vi "Everything.vi"() -> ()   [LabVIEW 2013]
uses:
  Version Token.ctl
  APU/Settings.ctl
  APU/Input.ctl
  APU/Output.ctl
  APU/Shared Settings.ctl
  Analog Replay/Settings.ctl
  Analog Replay/Input.ctl
  Analog Replay/Load Input.ctl
  Digital Pattern Generation/Load Input.ctl
  Digital Pattern Generation/Settings.ctl
  Digital Pattern Generation/Input.ctl
  ECU Event/Timing/Measure Output.ctl
  ECU Event/Timing/Measure Settings.ctl
  ECU Event/Timing/Capture Output.ctl
  Knock Sensor/Generate Input.ctl
  Knock Sensor/Cylinder Input.ctl
  Knock Sensor/Cylinder Settings.ctl
  Knock Sensor/Generate Settings.ctl
  Directional Speed/Load Input.ctl
  Directional Speed/Settings.ctl
  Directional Speed/Input.ctl
  <vilib>/Platform/TimedLoop/XDataNode/timing_clust.ctl
  <vilib>/Platform/TimedLoop/XDataNode/nitl_modes.ctl
  <vilib>/Platform/TimedLoop/XDataNode/wakeup.ctl
  ECU Event/Timing/Capture Settings.ctl
  <vilib>/rvi/DataTransferAndStorage/Container/Common/niFpgaContainerGetUniqueNameForEmu.vi
  <vilib>/rvi/DataTransferAndStorage/Container/Common/niFpgaContainerSetEmuInfo.vi
  <vilib>/rvi/eio/common/nirviEmuReportErrorAndStop.vi
  <vilib>/rvi/Emulation/niFpgaSctlEmulationGetInTimedLoop.vi
  <vilib>/rvi/Emulation/niFpgaEmulationReportErrorSimple.vi
  <vilib>/rvi/Emulation/niFpgaGetClockAttributes.vi
  <vilib>/rvi/Emulation/niFpgaCriticalErrorInLSC.vi
  <vilib>/rvi/eio/common/nirviEmuTemplateMethod_errors.vi
  ECU Event/Timing/Measure Events (40MHz).vi
  <vilib>/Platform/TimedLoop/XDataNode/XDataNode.xnode
  <vilib>/rvi/LocalResourceManager/LocalResourceManager.xnode
  <vilib>/eio/EIONode/EIONode.xnode
  APU/APU.lvlib
  <vilib>/Platform/TimedLoop/XDataNode/XDNodeRunTimeDep.lvlib
  Analog Replay/Analog Replay.lvlib
  Digital Pattern Generation/Digital Pattern Generation.lvlib
  ECU Event/Timing/ECU Event Timing.lvlib
  Knock Sensor/Knock Sensor.lvlib
  Directional Speed/Directional Speed.lvlib
  Engine Simulation Toolkit.lvlib
panel:
  in  "go.apu 1":bool
  in  "load input.Dir Speed DIO0":T1
  in  "input.Dir Speed DIO0":T2
  in  "settings.Dir Speed DIO0":T3
  in  "input.Dir Speed DIO1":T2
  in  "settings.Dir Speed DIO1":T3
  in  "load input.Dir Speed DIO1":T1
  in  "settings.Knock AO 3":T4
  in  "settings.Knock AO 3.Cylinder 1":T5
  in  "settings.Knock AO 3.Cylinder 2":T5
  in  "settings.Knock AO 3.Cylinder 3":T5
  in  "settings.Knock AO 3.Cylinder 4":T5
  in  "input.Knock AO 3.Cylinder 1":T6
  in  "input.Knock AO 3.Cylinder 2":T6
  in  "input.Knock AO 3.Cylinder 3":T6
  in  "input.Knock AO 3.Cylinder 4":T6
  in  "input.Knock AO 3":T7
  in  "settings.Knock AO 3.Cylinder 5":T5
  in  "settings.Knock AO 3.Cylinder 6":T5
  in  "input.Knock AO 3.Cylinder 5":T6
  in  "input.Knock AO 3.Cylinder 6":T6
  in  "settings.Knock AO 2.Cylinder 5":T5
  in  "settings.Knock AO 2.Cylinder 6":T5
  in  "input.Knock AO 2.Cylinder 5":T6={"probability compare"=65535, "high freq scaler"=0.0, "trigger position"=0}
  in  "input.Knock AO 2.Cylinder 6":T6={"probability compare"=65535, "high freq scaler"=0.0, "trigger position"=0}
  in  "settings.Knock AO 2":T4
  in  "settings.Knock AO 2.Cylinder 1":T5
  in  "settings.Knock AO 2.Cylinder 2":T5
  in  "settings.Knock AO 2.Cylinder 3":T5
  in  "settings.Knock AO 2.Cylinder 4":T5
  in  "input.Knock AO 2.Cylinder 1":T6={"probability compare"=65535, "high freq scaler"=0.0, "trigger position"=0}
  in  "input.Knock AO 2.Cylinder 2":T6={"probability compare"=65535, "high freq scaler"=0.0, "trigger position"=0}
  in  "input.Knock AO 2.Cylinder 3":T6={"probability compare"=65535, "high freq scaler"=0.0, "trigger position"=0}
  in  "input.Knock AO 2.Cylinder 4":T6={"probability compare"=65535, "high freq scaler"=0.0, "trigger position"=0}
  in  "input.Knock AO 2":T7
  out "capture.Multi Event DIO 15.Event 4":T8
  out "capture.Multi Event DIO 15.Event 3":T8
  out "capture.Multi Event DIO 15.Event 2":T8
  out "capture.Multi Event DIO 14.Event 4":T8
  out "capture.Multi Event DIO 14.Event 3":T8
  out "capture.Multi Event DIO 14.Event 2":T8
  out "capture.Multi Event DIO 13.Event 4":T8
  out "capture.Multi Event DIO 13.Event 3":T8
  out "capture.Multi Event DIO 13.Event 2":T8
  out "capture.Multi Event DIO 12.Event 4":T8
  out "capture.Multi Event DIO 12.Event 3":T8
  out "capture.Multi Event DIO 12.Event 2":T8
  out "capture.Multi Event DIO 11.Event 4":T8
  out "capture.Multi Event DIO 11.Event 3":T8
  out "capture.Multi Event DIO 11.Event 2":T8
  out "capture.Multi Event DIO 10.Event 4":T8
  out "capture.Multi Event DIO 10.Event 3":T8
  out "capture.Multi Event DIO 10.Event 2":T8
  out "capture.Multi Event DIO 10.Event 1":T8
  out "capture.Multi Event DIO 11.Event 1":T8
  out "capture.Multi Event DIO 12.Event 1":T8
  out "capture.Multi Event DIO 13.Event 1":T8
  out "capture.Multi Event DIO 14.Event 1":T8
  out "capture.Multi Event DIO 15.Event 1":T8
  in  "settings.Multi Event DIO 10":T9
  in  "settings.Multi Event DIO 11":T9
  in  "settings.Multi Event DIO 12":T9
  in  "settings.Multi Event DIO 13":T9
  in  "settings.Multi Event DIO 14":T9
  in  "settings.Multi Event DIO 15":T9
  out "status.Multi Event DIO 10":T10
  out "status.Multi Event DIO 11":T10
  out "status.Multi Event DIO 12":T10
  out "status.Multi Event DIO 13":T10
  out "status.Multi Event DIO 14":T10
  out "status.Multi Event DIO 15":T10
  out "capture.Event DIO 4.Event 1":T8
  out "capture.Event DIO 5.Event 1":T8
  out "capture.Event DIO 6.Event 1":T8
  out "capture.Event DIO 7.Event 1":T8
  out "capture.Event DIO 8.Event 1":T8
  out "capture.Event DIO 9.Event 1":T8
  in  "settings.Event DIO 4":T9
  in  "settings.Event DIO 5":T9
  in  "settings.Event DIO 6":T9
  in  "settings.Event DIO 7":T9
  in  "settings.Event DIO 8":T9
  in  "settings.Event DIO 9":T9
  out "status.Event DIO 4":T10
  out "status.Event DIO 5":T10
  out "status.Event DIO 6":T10
  out "status.Event DIO 7":T10
  out "status.Event DIO 8":T10
  out "status.Event DIO 9":T10
  in  "load input.Pattern DIO 3":T11
  in  "load input.Pattern DIO 2":T11
  in  "load input.Pattern DIO 1":T11
  in  "input.Pattern DIO 0":T12
  in  "settings.Pattern DIO 0":T13
  in  "input.Pattern DIO 1":T12
  in  "settings.Pattern DIO 1":T13
  in  "input.Pattern DIO 2":T12
  in  "settings.Pattern DIO 2":T13
  in  "input.Pattern DIO 3":T12
  in  "settings.Pattern DIO 3":T13
  in  "load input.Pattern DIO 0":T11
  in  "load input.replay AO 1":T14={"Data"=[0, 0, 0, 0, 0, 0, 0, 0, 0, 0, 0, 0, 0, 0, 0, 0], "LoadOffset"=0, "Done"=FALSE} caption="input"
  in  "load input.replay AO 0":T14={"Data"=[0, 0, 0, 0, 0, 0, 0, 0, 0, 0, 0, 0, 0, 0, 0, 0], "LoadOffset"=0, "Done"=FALSE} caption="input"
  in  "input.replay AO 0":T15 caption="input"
  in  "input.replay AO 1":T15 caption="input"
  in  "settings.replay AO 1":T16 caption="settings"
  in  "settings.replay AO 0":T16 caption="settings"
  in  "shared settings.apu 1":T17 {"start" format="%#.15g"}
  out "output.apu 1":T18 caption="output"
  in  "input.apu 1":T19={"desired speed"=0.0, "reset"=TRUE} caption="input"
  in  "settings.apu 1":T20 caption="settings"
  in  "est.version":T21
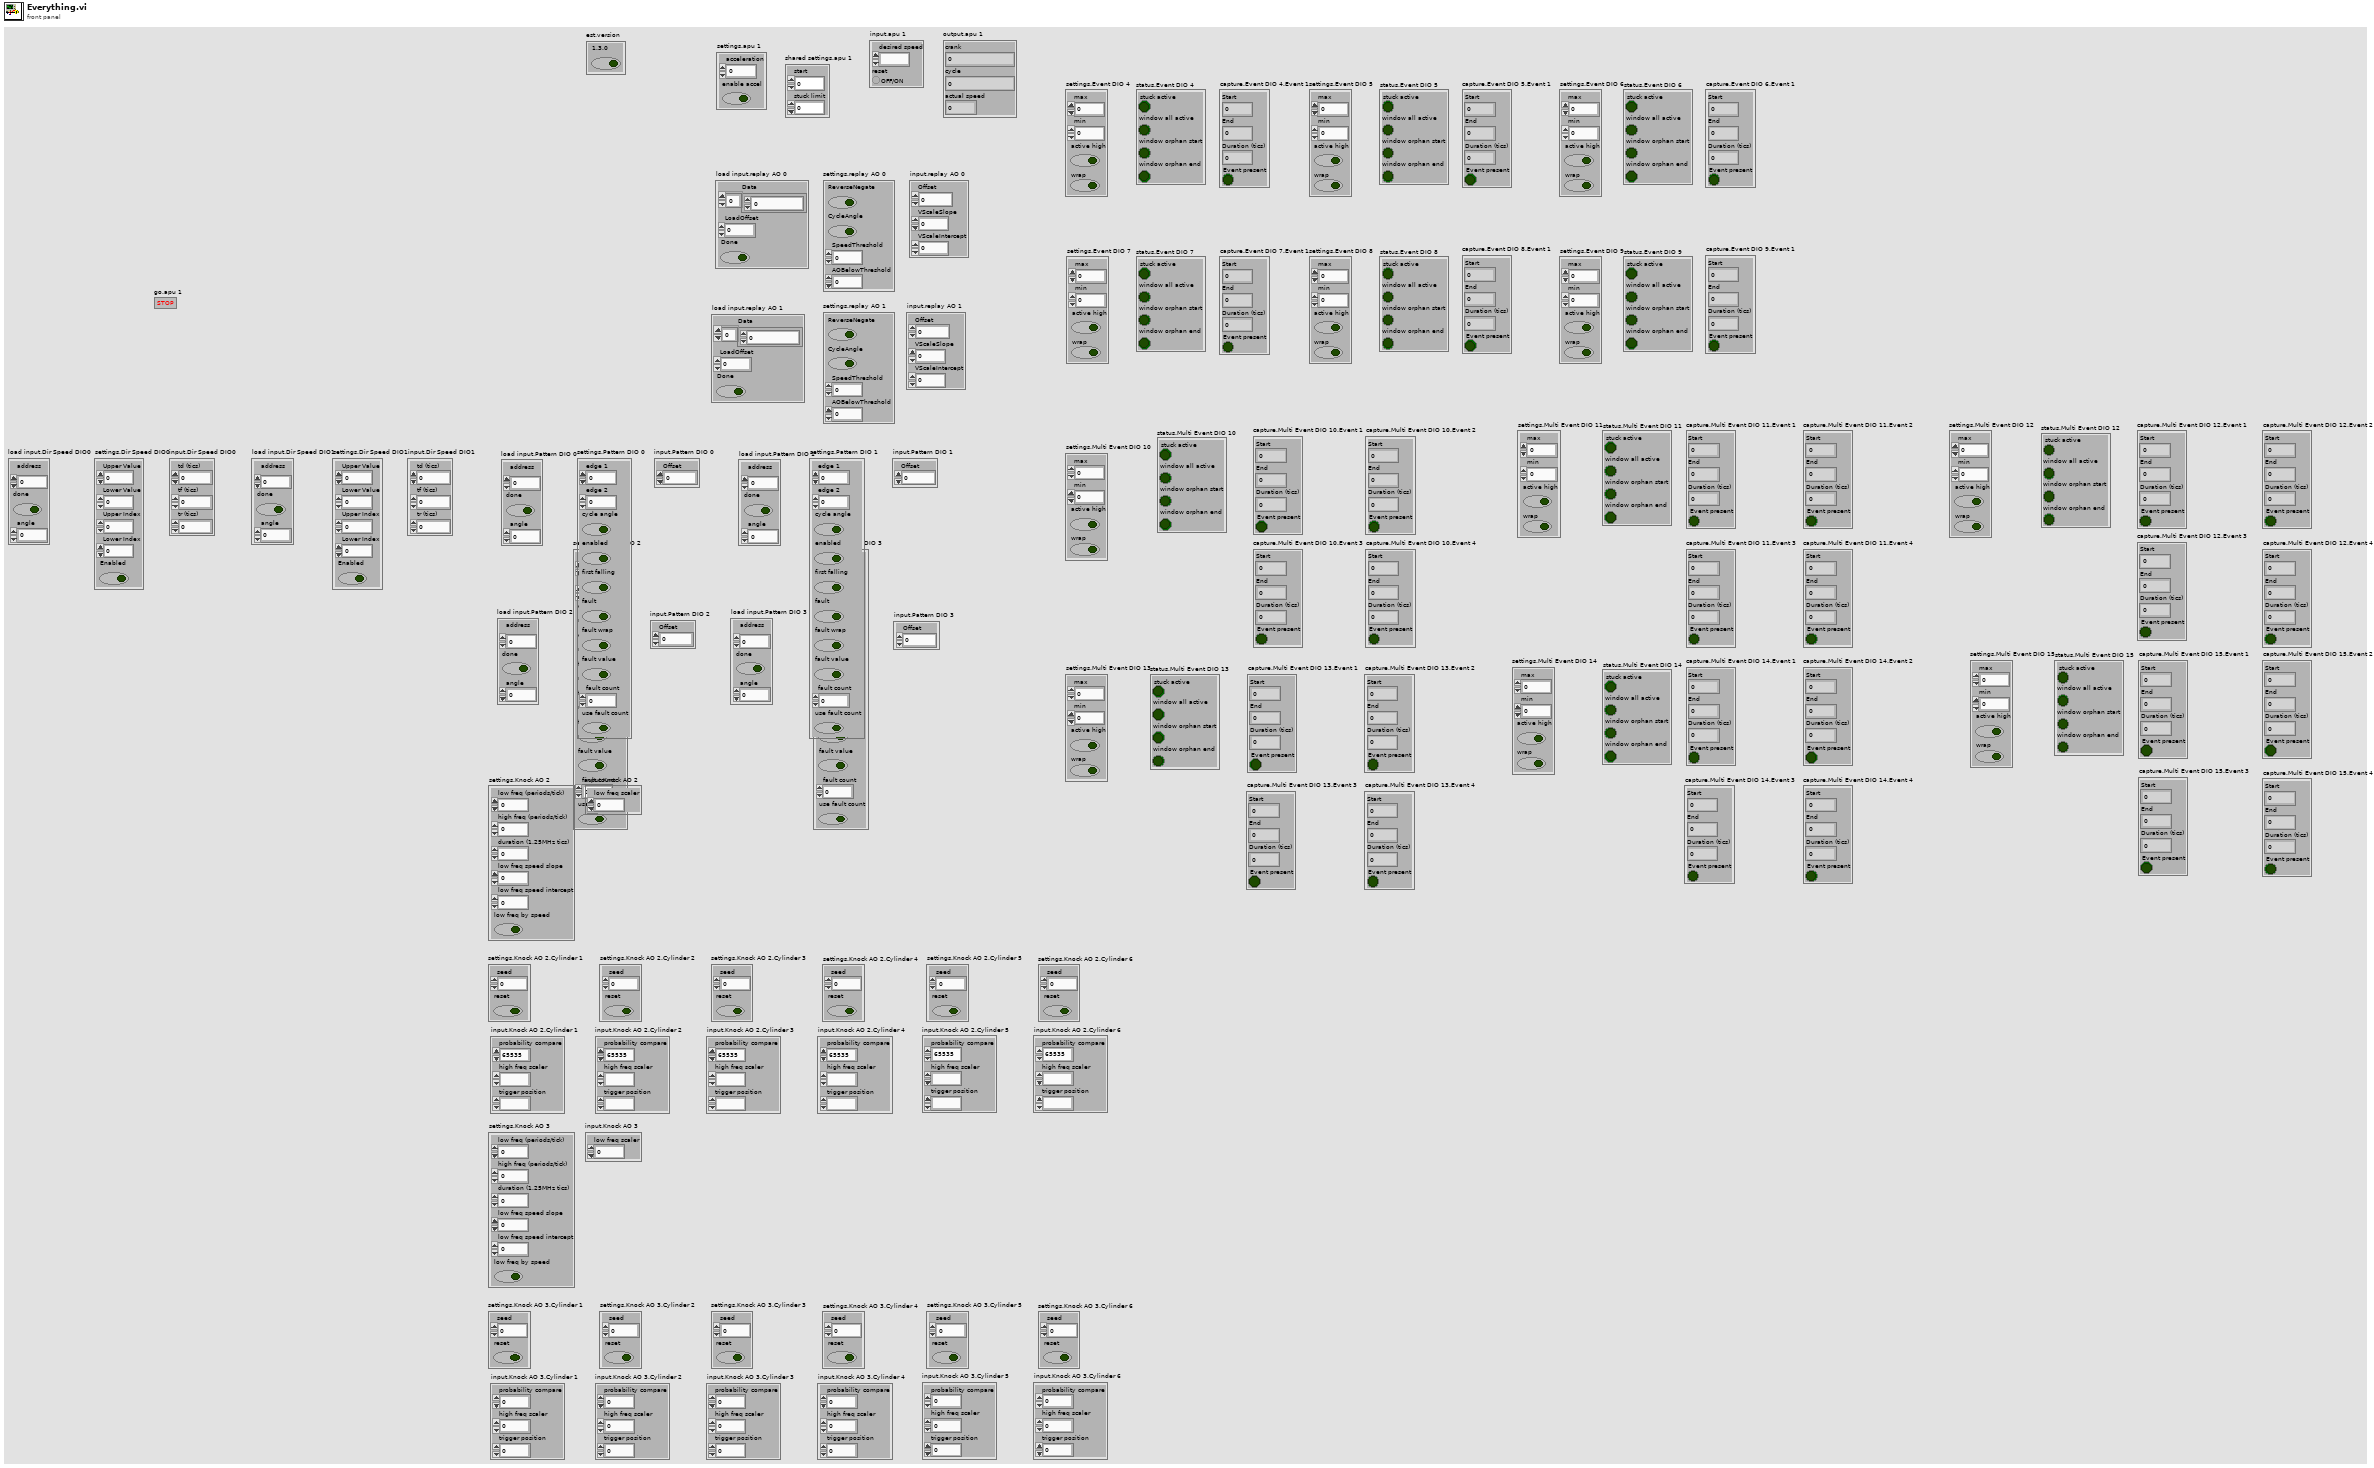
[diagram p1: front panel]
types:
  T1 = typedef "Engine Simulation Toolkit.lvlib/Directional Speed.lvlib/Load Input.ctl" = cluster{"address":fxp<+,10,10>, "done":bool, "angle":u16}
  T2 = typedef "Engine Simulation Toolkit.lvlib/Directional Speed.lvlib/Input.ctl" = cluster{"td (tics)":u16, "tf (tics)":u16, "tr (tics)":u16}
  T3 = typedef "Engine Simulation Toolkit.lvlib/Directional Speed.lvlib/Settings.ctl" = cluster{"Upper Value":u16, "Lower Value":u16, "Upper Index":fxp<+,10,10>, "Lower Index":fxp<+,10,10>, "Enabled":bool}
  T4 = typedef "Engine Simulation Toolkit.lvlib/Knock Sensor.lvlib/Generate Settings.ctl" = cluster{"low freq (periods/tick)":fxp<+,32,0>, "high freq (periods/tick)":fxp<+,32,0>, "duration (1.25MHz tics)":fxp<+,18,18>, "low freq speed slope":fxp<+,16,-3>, "low freq speed intercept":fxp<+,10,-10>, "low freq by speed":bool}
  T5 = typedef "Engine Simulation Toolkit.lvlib/Knock Sensor.lvlib/Cylinder Settings.ctl" = cluster{"seed":u16, "reset":bool}
  T6 = typedef "Engine Simulation Toolkit.lvlib/Knock Sensor.lvlib/Cylinder Input.ctl" = cluster{"probability compare":u16, "high freq scaler":fxp<+,10,0>, "trigger position":u16}
  T7 = typedef "Engine Simulation Toolkit.lvlib/Knock Sensor.lvlib/Generate Input.ctl" = cluster{"low freq scaler":fxp<+,10,0>}
  T8 = typedef "Engine Simulation Toolkit.lvlib/ECU Event Timing.lvlib/Capture Output.ctl" = cluster{"Start":u16, "End":u16, "Duration (tics)":fxp<+,18,18>, "Event present":bool}
  T9 = typedef "Engine Simulation Toolkit.lvlib/ECU Event Timing.lvlib/Measure Settings.ctl" = cluster{"max":u16, "min":u16, "active high":bool, "wrap":bool}
  T10 = typedef "Engine Simulation Toolkit.lvlib/ECU Event Timing.lvlib/Measure Output.ctl" = cluster{"stuck active":bool, "window all active":bool, "window orphan start":bool, "window orphan end":bool}
  T11 = typedef "Engine Simulation Toolkit.lvlib/Digital Pattern Generation.lvlib/Load Input.ctl" = cluster{"address":fxp<+,11,11>, "done":bool, "angle":u16}
  T12 = typedef "Engine Simulation Toolkit.lvlib/Digital Pattern Generation.lvlib/Input.ctl" = cluster{"Offset":i16}
  T13 = typedef "Engine Simulation Toolkit.lvlib/Digital Pattern Generation.lvlib/Settings.ctl" = cluster{"edge 1":u16, "edge 2":u16, "cycle angle":bool, "enabled":bool, "first falling":bool, "fault":bool, "fault wrap":bool, "fault value":bool, "fault count":fxp<+,4,4>, "use fault count":bool}
  T14 = typedef "Engine Simulation Toolkit.lvlib/Analog Replay.lvlib/Load Input.ctl" = cluster{"Data":i16[], "LoadOffset":u16, "Done":bool}
  T15 = typedef "Engine Simulation Toolkit.lvlib/Analog Replay.lvlib/Input.ctl" = cluster{"Offset":i16, "VScaleSlope":fxp<+,18,6>, "VScaleIntercept":fxp<+/-,18,3>}
  T16 = typedef "Engine Simulation Toolkit.lvlib/Analog Replay.lvlib/Settings.ctl" = cluster{"ReverseNegate":bool, "CycleAngle":bool, "SpeedThreshold":fxp<+/-,23,2>, "AOBelowThreshold":i16}
  T17 = typedef "Engine Simulation Toolkit.lvlib/APU.lvlib/Shared Settings.ctl" = cluster{"start":fxp<+,17,17>, "stuck limit":fxp<+,18,18>}
  T18 = typedef "Engine Simulation Toolkit.lvlib/APU.lvlib/Output.ctl" = cluster{"crank":u16, "cycle":u16, "actual speed":fxp<+/-,23,2>}
  T19 = typedef "Engine Simulation Toolkit.lvlib/APU.lvlib/Input.ctl" = cluster{"desired speed":fxp<+/-,23,2>, "reset":bool}
  T20 = typedef "Engine Simulation Toolkit.lvlib/APU.lvlib/Settings.ctl" = cluster{"acceleration":fxp<+,18,-20>, "enable accel":bool}
  T21 = typedef "Engine Simulation Toolkit.lvlib/Version Token.ctl" = cluster{"1.3.0":bool}
  T22 = typedef "XDNodeRunTimeDep.lvlib/timing_clust.ctl" = cluster{"Expected End [f-1]":u64, "Actual End [f-1]":u64, "Finished Late? [f-1]":bool, "Expected End [i-1]":u64, "Actual End [i-1]":u64, "Finished Late? [i-1]":bool, "Expected Start [i]":u64, "Actual Start [i]":u64, "Expected Start [f]":u64, "Actual Start [f]":u64, "Source Name":string, "Structure Name":string, "Period":i64, "Deadline":i64, "Offset":i64, "Start":i64, "Priority":i32, "Timeout":i32, "Mode":T23, "Wakeup Reason":T24, "Error":errorcluster, "Source Type":string, "Secondary Source Type":string, "Global End Time":u64, "Global Start Time":u64, "Frame Duration":u64, "Iteration Duration":u64, "Assigned CPU":i32, "I/O Scan Engine Mode":u32}
  T23 = typedef "XDNodeRunTimeDep.lvlib/nitl_modes.ctl" = enum32{"No Change", "Process missed periods, maintain original phase", "Discard missed periods, maintain original phase", "Process missed periods, ignore original phase", "Discard missed periods, ignore original phase"}
  T24 = typedef "XDNodeRunTimeDep.lvlib/wakeup.ctl" = enum32{"Normal", "Aborted", "Asynchronous wakeup", "Timing source error", "Timed loop error", "Timeout"}
  T25 = typedef "Engine Simulation Toolkit.lvlib/Directional Speed.lvlib/Load Data.ctl" = cluster{"max address":fxp<+,10,10>, "Memory":refnum<k21>}
  T26 = typedef "Engine Simulation Toolkit.lvlib/APU.lvlib/Register Bus.ctl" = cluster{"Speed":refnum<k21>, "Crank Angle":refnum<k21>, "Cycle Angle":refnum<k21>, "Crank Count":refnum<k21>, "Cycle Count":refnum<k21>, "1.25 MHz Counter":refnum<k21>, "Crank Rollover":refnum<k21>, "Cycle Rollover":refnum<k21>, "shared settings":T17}
  T27 = typedef "Engine Simulation Toolkit.lvlib/Digital Pattern Generation.lvlib/Load Data.ctl" = cluster{"max address":fxp<+,11,11>, "memory":refnum<k21>}
  T28 = typedef "Engine Simulation Toolkit.lvlib/Knock Sensor.lvlib/Triggered Cylinder Data.ctl" = cluster{"trigger knock":bool, "high freq scaler":fxp<+,10,0>}
  T29 = typedef "Engine Simulation Toolkit.lvlib/ECU Event Timing.lvlib/Capture Settings.ctl" = u8
  T30 = typedef "Engine Simulation Toolkit.lvlib/ECU Event Timing.lvlib/Measured Data.ctl" = cluster{"start":u16, "end":u16, "duration (tics)":fxp<+,18,18>, "window end":bool, "window begin":bool, "pulse end":bool, "pulse #":u8}
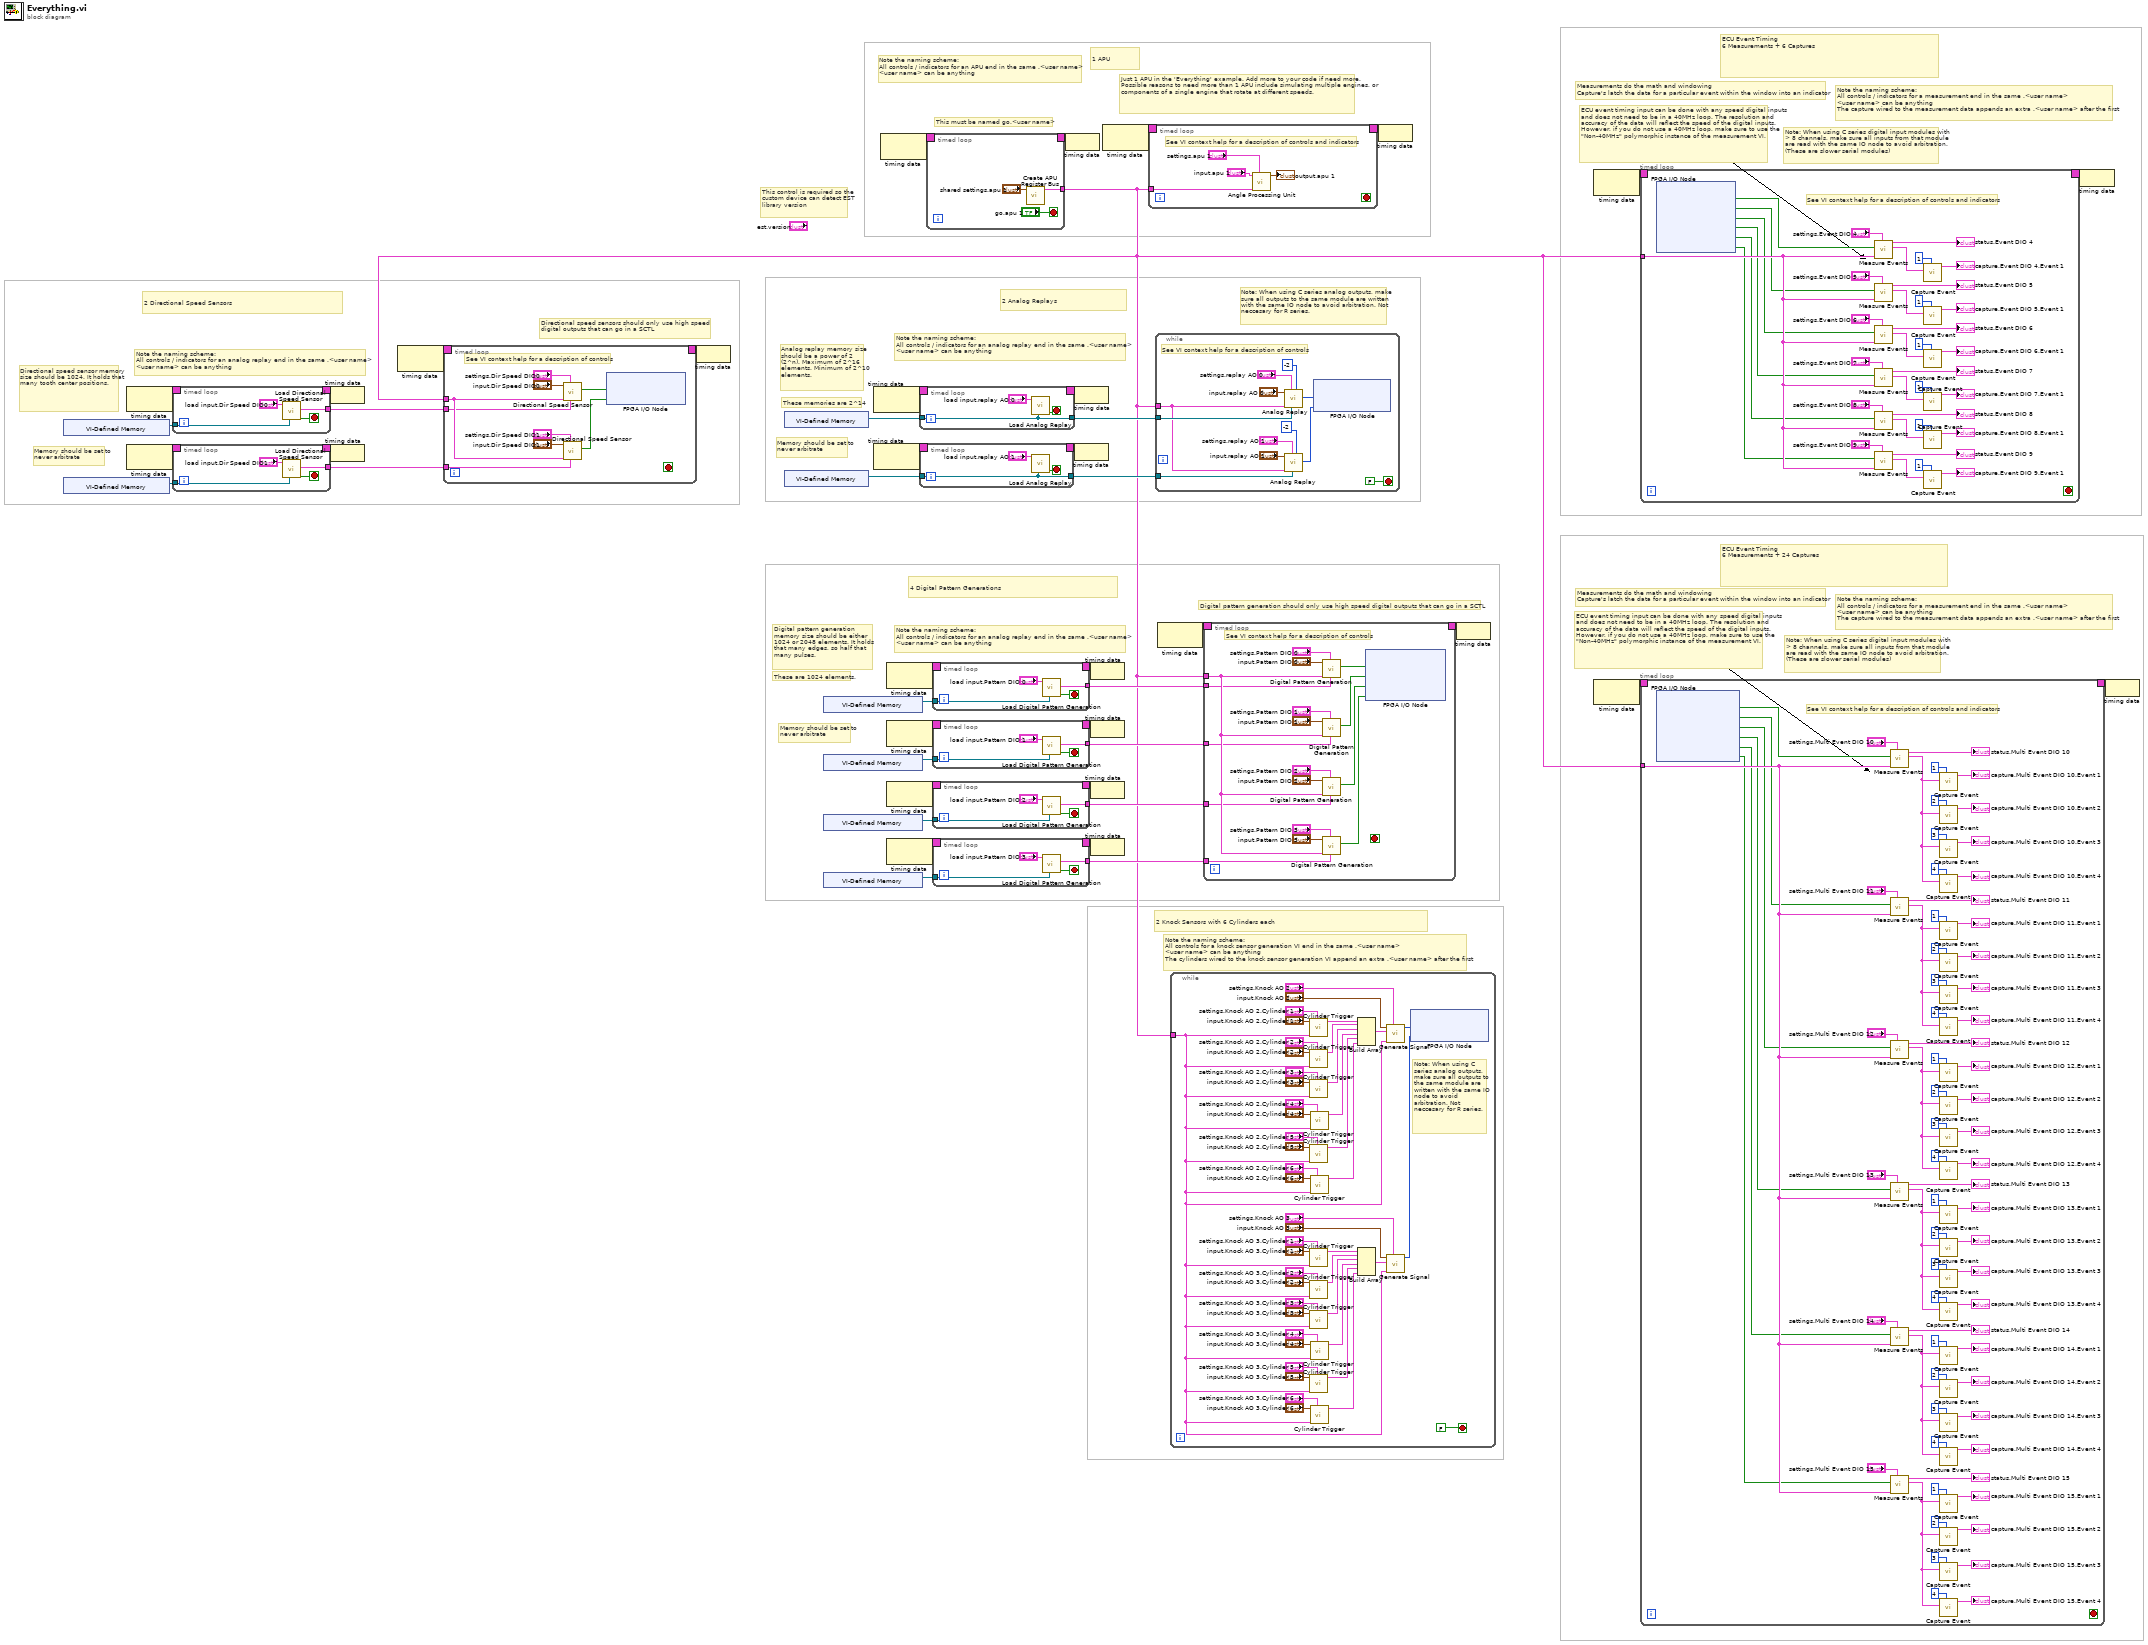
[diagram p0: block diagram]
diagram:
  # "ECU event timing input can be done with any speed digital inputs and does not need to be in a 40MHz loop. The resolution and accuracy of the data will reflect the speed of the digital inputs. However, if you do not use a 40MHz loop, make sure to use the \"Non-40MHz\" polymorphic instance of the measurement VI."
  # "This must be named go.<user name>"
  # "Memory should be set to never arbitrate"
  # "Memory should be set to never arbitrate"
  # "Memory should be set to never arbitrate"
  # "Note the naming scheme: \nAll controls / indicators for an analog replay end in the same .<user name>\n<user name> can be anything"
  # "Directional speed sensor memory size should be 1024. It holds that many tooth center positions."
  # "Directional speed sensors should only use high speed digital outputs that can go in a SCTL"
  # "2 Directional Speed Sensors"
  # "Note the naming scheme: \nAll controls for a knock sensor generation VI end in the same .<user name>\n<user name> can be anything\nThe cylinders wired to the knock sensor generation VI append an extra .<user name> after the first"
  # "2 Knock Sensors with 6 Cylinders each"
  # "Note: When using C series digital input modules with > 8 channels, make sure all inputs from that module are read with the same IO node to avoid arbitration. (These are slower serial modules)"
  # "Measurements do the math and windowing\nCapture's latch the data for a particular event within the window into an indicator"
  # "ECU Event Timing\n6 Measurements + 24 Captures"
  # "Note the naming scheme: \nAll controls / indicators for a measurement end in the same .<user name>\n<user name> can be anything\nThe capture wired to the measurement data appends an extra .<user name> after the first"
  # "Note: When using C series digital input modules with > 8 channels, make sure all inputs from that module are read with the same IO node to avoid arbitration. (These are slower serial modules)"
  # "Measurements do the math and windowing\nCapture's latch the data for a particular event within the window into an indicator"
  # "ECU Event Timing\n6 Measurements + 6 Captures"
  # "Note the naming scheme: \nAll controls / indicators for a measurement end in the same .<user name>\n<user name> can be anything\nThe capture wired to the measurement data appends an extra .<user name> after the first"
  # "ECU event timing input can be done with any speed digital inputs and does not need to be in a 40MHz loop. The resolution and accuracy of the data will reflect the speed of the digital inputs. However, if you do not use a 40MHz loop, make sure to use the \"Non-40MHz\" polymorphic instance of the measurement VI."
  # "Digital pattern generation should only use high speed digital outputs that can go in a SCTL"
  # "4 Digital Pattern Generations"
  # "Note the naming scheme: \nAll controls / indicators for an analog replay end in the same .<user name>\n<user name> can be anything"
  # "These are 1024 elements."
  # "Digital pattern generation memory size should be either 1024 or 2048 elements. It holds that many edges, so half that many pulses."
  # "Note: When using C series analog outputs, make sure all outputs to the same module are written with the same IO node to avoid arbitration. Not neccesary for R series."
  # "2 Analog Replays"
  # "1 APU"
  # "These memories are 2^14"
  # "Note the naming scheme: \nAll controls / indicators for an APU end in the same .<user name>\n<user name> can be anything"
  # "Note the naming scheme: \nAll controls / indicators for an analog replay end in the same .<user name>\n<user name> can be anything"
  # "Analog replay memory size should be a power of 2 (2^n). Maximum of 2^16 elements. Minimum of 2^10 elements."
  # "Just 1 APU in the 'Everything' example. Add more to your code if need more. Possible reasons to need more than 1 APU include simulating multiple engines, or components of a single engine that rotate at different speeds."
  # "This control is required so the custom device can detect EST library version"
  n1 = xnode "VI-Defined Memory"() -> ("Memory Out"=w4:refnum<k21>)
  n2 = xnode "VI-Defined Memory"() -> ("Memory Out"=w6:refnum<k21>)
  n3 = node-c288() -> (w13:T22)  [unwired: 1 in]
  n4 = node-c288() -> (w9:T22)  [unwired: 1 in]
  n5 = timed-loop {
    timing: w13 -> [_]
    timing-out: [_] -> w12
    tunnel: w4 -> [w48]
    tunnel: [w47] -> w5
    stop <- w49 stop-if-true
    n6 = call "Load Directional Speed Sensor.vi"("Memory In"=w48, "load input.<user name>"="load input.Dir Speed DIO0") -> ("done"=w49:bool, "load data"=w47:T25)  [unwired: 8 in]
  }
  n7 = timed-loop {
    timing: w9 -> [_]
    timing-out: [_] -> w8
    tunnel: w6 -> [w54]
    tunnel: [w53] -> w7
    stop <- w55 stop-if-true
    n8 = call "Load Directional Speed Sensor.vi"("Memory In"=w54, "load input.<user name>"="load input.Dir Speed DIO1") -> ("done"=w55:bool, "load data"=w53:T25)  [unwired: 8 in]
  }
  n9 = node-c288(w12) -> ()
  n10 = node-c288(w8) -> ()
  n11 = node-c288() -> (w11:T22)  [unwired: 1 in]
  n12 = xnode "VI-Defined Memory"() -> ("Memory Out"=w38:refnum<k21>)
  n13 = xnode "VI-Defined Memory"() -> ("Memory Out"=w39:refnum<k21>)
  n14 = xnode "VI-Defined Memory"() -> ("Memory Out"=w31:refnum<k21>)
  n15 = xnode "VI-Defined Memory"() -> ("Memory Out"=w27:refnum<k21>)
  n16 = xnode "VI-Defined Memory"() -> ("Memory Out"=w24:refnum<k21>)
  n17 = xnode "VI-Defined Memory"() -> ("Memory Out"=w21:refnum<k21>)
  n18 = node-c288() -> (w43:T22)  [unwired: 1 in]
  n19 = node-c288() -> (w41:T22)  [unwired: 1 in]
  n20 = node-c288() -> (w2:T22)  [unwired: 1 in]
  n21 = node-c288() -> (w35:T22)  [unwired: 1 in]
  n22 = node-c288() -> (w29:T22)  [unwired: 1 in]
  n23 = node-c288() -> (w26:T22)  [unwired: 1 in]
  n24 = node-c288() -> (w23:T22)  [unwired: 1 in]
  n25 = timed-loop {
    timing: w43 -> [_]
    timing-out: [_] -> w42
    tunnel: w38 -> [w58]
    tunnel: [w58] -> w37
    stop <- w59 stop-if-true
    n26 = call "Load Analog Replay.vi"("memory"=w58, "load input.<user name>"="load input.replay AO 0") -> ("done"=w59:bool)  [unwired: 9 in]
  }
  n27 = timed-loop {
    timing: w41 -> [_]
    timing-out: [_] -> w40
    tunnel: w39 -> [w63]
    tunnel: [w63] -> w36
    stop <- w64 stop-if-true
    n28 = call "Load Analog Replay.vi"("memory"=w63, "load input.<user name>"="load input.replay AO 1") -> ("done"=w64:bool)  [unwired: 9 in]
  }
  n29 = timed-loop {
    timing: w2 -> [_]
    timing-out: [_] -> w1
    tunnel: [w69] -> w3
    stop <- "go.apu 1" stop-if-true
    n30 = call "Create APU Register Bus.vi"("shared settings.<user name>"="shared settings.apu 1") -> ("register bus"=w69:T26)  [unwired: 10 in]
  }
  n31 = timed-loop {
    tunnel: w3 -> [w75]
    timing: w11 -> [_]
    timing-out: [_] -> w10
    tunnel: w5 -> [w74]
    tunnel: w7 -> [w73]
    stop <- _ stop-if-true
    # "See VI context help for a description of controls"
    n32 = call "Directional Speed Sensor.vi"("load data"=w74, "settings.<user name>"="settings.Dir Speed DIO0", "register bus"=w75, "input.<user name>"="input.Dir Speed DIO0") -> ("digial output"=w78:bool)  [unwired: 7 in]
    n33 = call "Directional Speed Sensor.vi"("load data"=w73, "settings.<user name>"="settings.Dir Speed DIO1", "register bus"=w75, "input.<user name>"="input.Dir Speed DIO1") -> ("digial output"=w79:bool)  [unwired: 7 in]
    n34 = xnode "FPGA I/O Node"("Connector1/DIO0"=w78, "Connector1/DIO1"=w79) -> ()  [unwired: 2 in, 2 out]
  }
  n35 = node-c288(w10) -> ()
  n36 = timed-loop {
    timing: w35 -> [_]
    timing-out: [_] -> w34
    tunnel: w31 -> [w86]
    tunnel: [w85] -> w30
    stop <- w87 stop-if-true
    n37 = call "Load Digital Pattern Generation.vi"("memory"=w86, "load input.<user name>"="load input.Pattern DIO 0") -> ("done"=w87:bool, "load data"=w85:T27)  [unwired: 8 in]
  }
  n38 = timed-loop {
    timing: w29 -> [_]
    timing-out: [_] -> w28
    tunnel: w27 -> [w92]
    tunnel: [w91] -> w18
    stop <- w93 stop-if-true
    n39 = call "Load Digital Pattern Generation.vi"("memory"=w92, "load input.<user name>"="load input.Pattern DIO 1") -> ("done"=w93:bool, "load data"=w91:T27)  [unwired: 8 in]
  }
  n40 = timed-loop {
    timing: w26 -> [_]
    timing-out: [_] -> w25
    tunnel: w24 -> [w98]
    tunnel: [w97] -> w19
    stop <- w99 stop-if-true
    n41 = call "Load Digital Pattern Generation.vi"("memory"=w98, "load input.<user name>"="load input.Pattern DIO 2") -> ("done"=w99:bool, "load data"=w97:T27)  [unwired: 8 in]
  }
  n42 = timed-loop {
    timing: w23 -> [_]
    timing-out: [_] -> w22
    tunnel: w21 -> [w104]
    tunnel: [w103] -> w20
    stop <- w105 stop-if-true
    n43 = call "Load Digital Pattern Generation.vi"("memory"=w104, "load input.<user name>"="load input.Pattern DIO 3") -> ("done"=w105:bool, "load data"=w103:T27)  [unwired: 8 in]
  }
  n44 = node-c288(w1) -> ()
  n45 = node-c288(w40) -> ()
  n46 = node-c288(w42) -> ()
  n47 = node-c288(w34) -> ()
  n48 = node-c288(w28) -> ()
  n49 = node-c288(w25) -> ()
  n50 = node-c288(w22) -> ()
  n51 = node-c288() -> (w45:T22)  [unwired: 1 in]
  n52 = timed-loop {
    timing: w45 -> [_]
    timing-out: [_] -> w44
    tunnel: w3 -> [w108]
    stop <- _ stop-if-true
    # "See VI context help for a description of controls and indicators"
    n53 = call "Angle Processing Unit.vi"("settings.<user name>"="settings.apu 1", "register bus"=w108, "input.<user name>"="input.apu 1") -> ("output.<user name>"=→"output.apu 1":T18)  [unwired: 8 in]
  }
  n54 = while {
    tunnel: w37 -> [w125]
    tunnel: w3 -> [w114]
    tunnel: w36 -> [w122]
    stop <- FALSE stop-if-true
    # "See VI context help for a description of controls"
    n55 = call "Analog Replay.vi"("shift"=i8 -2, "memory"=w125, "settings.<user name>"="settings.replay AO 0", "register bus"=w114, "input.<user name>"="input.replay AO 0") -> ("analog value"=w118:i16)  [unwired: 6 in]
    n56 = call "Analog Replay.vi"("shift"=i8 -2, "memory"=w122, "settings.<user name>"="settings.replay AO 1", "register bus"=w114, "input.<user name>"="input.replay AO 1") -> ("analog value"=w117:i16)  [unwired: 6 in]
    n57 = xnode "FPGA I/O Node"("Connector0/AO0"=w118, "Connector0/AO1"=w117) -> ()  [unwired: 2 in, 2 out]
  }
  n58 = node-c288() -> (w33:T22)  [unwired: 1 in]
  n59 = while {
    tunnel: w3 -> [w127]
    stop <- FALSE stop-if-true
    # "Note: When using C series analog outputs, make sure all outputs to the same module are written with the same IO node to avoid arbitration. Not neccesary for R series."
    n60 = call "Cylinder Trigger.vi"("settings.<user name>"="settings.Knock AO 2.Cylinder 1", "register bus"=w127, "input.<user name>"="input.Knock AO 2.Cylinder 1") -> ("triggered knock data"=w171:T28)  [unwired: 8 in]
    n61 = call "Cylinder Trigger.vi"("settings.<user name>"="settings.Knock AO 2.Cylinder 2", "register bus"=w127, "input.<user name>"="input.Knock AO 2.Cylinder 2") -> ("triggered knock data"=w170:T28)  [unwired: 8 in]
    n62 = call "Cylinder Trigger.vi"("settings.<user name>"="settings.Knock AO 2.Cylinder 3", "register bus"=w127, "input.<user name>"="input.Knock AO 2.Cylinder 3") -> ("triggered knock data"=w169:T28)  [unwired: 8 in]
    n63 = call "Cylinder Trigger.vi"("settings.<user name>"="settings.Knock AO 2.Cylinder 5", "register bus"=w127, "input.<user name>"="input.Knock AO 2.Cylinder 5") -> ("triggered knock data"=w150:T28)  [unwired: 8 in]
    n64 = call "Cylinder Trigger.vi"("settings.<user name>"="settings.Knock AO 3.Cylinder 1", "register bus"=w127, "input.<user name>"="input.Knock AO 3.Cylinder 1") -> ("triggered knock data"=w128:T28)  [unwired: 8 in]
    n65 = call "Cylinder Trigger.vi"("settings.<user name>"="settings.Knock AO 3.Cylinder 2", "register bus"=w127, "input.<user name>"="input.Knock AO 3.Cylinder 2") -> ("triggered knock data"=w129:T28)  [unwired: 8 in]
    n66 = call "Cylinder Trigger.vi"("settings.<user name>"="settings.Knock AO 3.Cylinder 3", "register bus"=w127, "input.<user name>"="input.Knock AO 3.Cylinder 3") -> ("triggered knock data"=w130:T28)  [unwired: 8 in]
    n67 = call "Cylinder Trigger.vi"("settings.<user name>"="settings.Knock AO 3.Cylinder 5", "register bus"=w127, "input.<user name>"="input.Knock AO 3.Cylinder 5") -> ("triggered knock data"=w147:T28)  [unwired: 8 in]
    n68 = call "Cylinder Trigger.vi"("settings.<user name>"="settings.Knock AO 2.Cylinder 4", "register bus"=w127, "input.<user name>"="input.Knock AO 2.Cylinder 4") -> ("triggered knock data"=w168:T28)  [unwired: 8 in]
    n69 = call "Cylinder Trigger.vi"("settings.<user name>"="settings.Knock AO 2.Cylinder 6", "register bus"=w127, "input.<user name>"="input.Knock AO 2.Cylinder 6") -> ("triggered knock data"=w149:T28)  [unwired: 8 in]
    n70 = call "Cylinder Trigger.vi"("settings.<user name>"="settings.Knock AO 3.Cylinder 4", "register bus"=w127, "input.<user name>"="input.Knock AO 3.Cylinder 4") -> ("triggered knock data"=w131:T28)  [unwired: 8 in]
    n71 = call "Cylinder Trigger.vi"("settings.<user name>"="settings.Knock AO 3.Cylinder 6", "register bus"=w127, "input.<user name>"="input.Knock AO 3.Cylinder 6") -> ("triggered knock data"=w148:T28)  [unwired: 8 in]
    n72 = Build Array(w171, w170, w169, w168, w150, w149) -> (w167:T28[])
    n73 = Build Array(w128, w129, w130, w131, w147, w148) -> (w132:T28[])
    n74 = call "Generate Signal.vi"("settings.<user name>"="settings.Knock AO 2", "register bus"=w127, "triggered knock data"=w167, "input.<user name>"="input.Knock AO 2") -> ("knock signal"=w155:i16)  [unwired: 7 in]
    n75 = call "Generate Signal.vi"("settings.<user name>"="settings.Knock AO 3", "register bus"=w127, "triggered knock data"=w132, "input.<user name>"="input.Knock AO 3") -> ("knock signal"=w126:i16)  [unwired: 7 in]
    n76 = xnode ("FPGA I/O Node")("Connector0/AO2"=w155, "Connector0/AO3"=w126) -> ()  [unwired: 2 in, 2 out]
  }
  n77 = timed-loop {
    tunnel: w3 -> [w176]
    timing: w33 -> [_]
    timing-out: [_] -> w32
    tunnel: w30 -> [w175]
    tunnel: w18 -> [w174]
    tunnel: w19 -> [w173]
    tunnel: w20 -> [w172]
    stop <- _ stop-if-true
    # "See VI context help for a description of controls"
    n78 = call "Digital Pattern Generation.vi"("load data"=w175, "settings.<user name>"="settings.Pattern DIO 0", "register bus"=w176, "input.<user name>"="input.Pattern DIO 0") -> ("digial output"=w181:bool)  [unwired: 7 in]
    n79 = call "Digital Pattern Generation.vi"("load data"=w174, "settings.<user name>"="settings.Pattern DIO 1", "register bus"=w176, "input.<user name>"="input.Pattern DIO 1") -> ("digial output"=w182:bool)  [unwired: 7 in]
    n80 = call "Digital Pattern Generation.vi"("load data"=w173, "settings.<user name>"="settings.Pattern DIO 2", "register bus"=w176, "input.<user name>"="input.Pattern DIO 2") -> ("digial output"=w183:bool)  [unwired: 7 in]
    n81 = call "Digital Pattern Generation.vi"("load data"=w172, "settings.<user name>"="settings.Pattern DIO 3", "register bus"=w176, "input.<user name>"="input.Pattern DIO 3") -> ("digial output"=w184:bool)  [unwired: 7 in]
    n82 = xnode "FPGA I/O Node"("Connector0/DIO0"=w181, "Connector0/DIO1"=w182, "Connector0/DIO2"=w183, "Connector0/DIO3"=w184) -> ()  [unwired: 4 in, 4 out]
  }
  n83 = node-c288(w44) -> ()
  n84 = node-c288(w32) -> ()
  n85 = node-c288() -> (w17:T22)  [unwired: 1 in]
  n86 = node-c288() -> (w15:T22)  [unwired: 1 in]
  n87 = timed-loop {
    timing: w17 -> [_]
    timing-out: [_] -> w16
    tunnel: w3 -> [w221]
    stop <- _ stop-if-true
    # "See VI context help for a description of controls and indicators"
    n88 = xnode "FPGA I/O Node"() -> ("Connector0/DIO4"=w202:bool, "Connector0/DIO5"=w201:bool, "Connector0/DIO6"=w200:bool, "Connector0/DIO7"=w199:bool, "Connector0/DIO8"=w198:bool, "Connector0/DIO9"=w197:bool)  [unwired: 6 in, 6 out]
    n89 = call-poly "Measure Events.vi"("settings.<user name>"="settings.Event DIO 4", "register bus"=w221, "event"=w202) -> ("measured data"=w220:T30, "status.<user name>"=→"status.Event DIO 4":T10)  [unwired: 7 in]
    n90 = call-poly "Measure Events.vi"("settings.<user name>"="settings.Event DIO 5", "register bus"=w221, "event"=w201) -> ("measured data"=w213:T30, "status.<user name>"=→"status.Event DIO 5":T10)  [unwired: 7 in]
    n91 = call-poly "Measure Events.vi"("settings.<user name>"="settings.Event DIO 6", "register bus"=w221, "event"=w200) -> ("measured data"=w212:T30, "status.<user name>"=→"status.Event DIO 6":T10)  [unwired: 7 in]
    n92 = call-poly "Measure Events.vi"("settings.<user name>"="settings.Event DIO 7", "register bus"=w221, "event"=w199) -> ("measured data"=w211:T30, "status.<user name>"=→"status.Event DIO 7":T10)  [unwired: 7 in]
    n93 = call-poly "Measure Events.vi"("settings.<user name>"="settings.Event DIO 8", "register bus"=w221, "event"=w198) -> ("measured data"=w210:T30, "status.<user name>"=→"status.Event DIO 8":T10)  [unwired: 7 in]
    n94 = call-poly "Measure Events.vi"("settings.<user name>"="settings.Event DIO 9", "register bus"=w221, "event"=w197) -> ("measured data"=w209:T30, "status.<user name>"=→"status.Event DIO 9":T10)  [unwired: 7 in]
    n95 = call "Capture Event.vi"("event # to capture"=T29 1 ("Settings.spark 1 shot 1"), "measured data"=w220) -> ("capture.<user name>"=→"capture.Event DIO 4.Event 1":T8)  [unwired: 9 in]
    n96 = call "Capture Event.vi"("event # to capture"=T29 1 ("Settings.spark 2 shot 1"), "measured data"=w213) -> ("capture.<user name>"=→"capture.Event DIO 5.Event 1":T8)  [unwired: 9 in]
    n97 = call "Capture Event.vi"("event # to capture"=T29 1 ("Settings.spark 3 shot 1"), "measured data"=w212) -> ("capture.<user name>"=→"capture.Event DIO 6.Event 1":T8)  [unwired: 9 in]
    n98 = call "Capture Event.vi"("event # to capture"=T29 1 ("Settings.spark 4 shot 1"), "measured data"=w211) -> ("capture.<user name>"=→"capture.Event DIO 7.Event 1":T8)  [unwired: 9 in]
    n99 = call "Capture Event.vi"("event # to capture"=T29 1 ("Settings.spark 5 shot 1"), "measured data"=w210) -> ("capture.<user name>"=→"capture.Event DIO 8.Event 1":T8)  [unwired: 9 in]
    n100 = call "Capture Event.vi"("event # to capture"=T29 1 ("Settings.spark 6 shot 1"), "measured data"=w209) -> ("capture.<user name>"=→"capture.Event DIO 9.Event 1":T8)  [unwired: 9 in]
  }
  n101 = timed-loop {
    timing: w15 -> [_]
    timing-out: [_] -> w14
    tunnel: w3 -> [w296]
    stop <- _ stop-if-true
    # "See VI context help for a description of controls and indicators"
    n102 = xnode "FPGA I/O Node"() -> ("Connector0/DIO10"=w283:bool, "Connector0/DIO11"=w282:bool, "Connector0/DIO12"=w281:bool, "Connector0/DIO13"=w280:bool, "Connector0/DIO14"=w279:bool, "Connector0/DIO15"=w278:bool)  [unwired: 6 in, 6 out]
    n103 = call-poly "Measure Events.vi"("settings.<user name>"="settings.Multi Event DIO 10", "register bus"=w296, "event"=w283) -> ("measured data"=w265:T30, "status.<user name>"=→"status.Multi Event DIO 10":T10)  [unwired: 7 in]
    n104 = call-poly "Measure Events.vi"("settings.<user name>"="settings.Multi Event DIO 11", "register bus"=w296, "event"=w282) -> ("measured data"=w258:T30, "status.<user name>"=→"status.Multi Event DIO 11":T10)  [unwired: 7 in]
    n105 = call-poly "Measure Events.vi"("settings.<user name>"="settings.Multi Event DIO 12", "register bus"=w296, "event"=w281) -> ("measured data"=w251:T30, "status.<user name>"=→"status.Multi Event DIO 12":T10)  [unwired: 7 in]
    n106 = call-poly "Measure Events.vi"("settings.<user name>"="settings.Multi Event DIO 13", "register bus"=w296, "event"=w280) -> ("measured data"=w244:T30, "status.<user name>"=→"status.Multi Event DIO 13":T10)  [unwired: 7 in]
    n107 = call-poly "Measure Events.vi"("settings.<user name>"="settings.Multi Event DIO 14", "register bus"=w296, "event"=w279) -> ("measured data"=w237:T30, "status.<user name>"=→"status.Multi Event DIO 14":T10)  [unwired: 7 in]
    n108 = call-poly "Measure Events.vi"("settings.<user name>"="settings.Multi Event DIO 15", "register bus"=w296, "event"=w278) -> ("measured data"=w230:T30, "status.<user name>"=→"status.Multi Event DIO 15":T10)  [unwired: 7 in]
    n109 = call "Capture Event.vi"("event # to capture"=T29 1 ("Settings.spark 1 shot 1"), "measured data"=w265) -> ("capture.<user name>"=→"capture.Multi Event DIO 10.Event 1":T8)  [unwired: 9 in]
    n110 = call "Capture Event.vi"("event # to capture"=T29 2 ("Settings.spark 1 shot 1"), "measured data"=w265) -> ("capture.<user name>"=→"capture.Multi Event DIO 10.Event 2":T8)  [unwired: 9 in]
    n111 = call "Capture Event.vi"("event # to capture"=T29 3 ("Settings.spark 1 shot 1"), "measured data"=w265) -> ("capture.<user name>"=→"capture.Multi Event DIO 10.Event 3":T8)  [unwired: 9 in]
    n112 = call "Capture Event.vi"("event # to capture"=T29 4 ("Settings.spark 1 shot 1"), "measured data"=w265) -> ("capture.<user name>"=→"capture.Multi Event DIO 10.Event 4":T8)  [unwired: 9 in]
    n113 = call "Capture Event.vi"("event # to capture"=T29 1 ("Settings.spark 2 shot 1"), "measured data"=w258) -> ("capture.<user name>"=→"capture.Multi Event DIO 11.Event 1":T8)  [unwired: 9 in]
    n114 = call "Capture Event.vi"("event # to capture"=T29 2 ("Settings.spark 2 shot 1"), "measured data"=w258) -> ("capture.<user name>"=→"capture.Multi Event DIO 11.Event 2":T8)  [unwired: 9 in]
    n115 = call "Capture Event.vi"("event # to capture"=T29 3 ("Settings.spark 2 shot 1"), "measured data"=w258) -> ("capture.<user name>"=→"capture.Multi Event DIO 11.Event 3":T8)  [unwired: 9 in]
    n116 = call "Capture Event.vi"("event # to capture"=T29 4 ("Settings.spark 2 shot 1"), "measured data"=w258) -> ("capture.<user name>"=→"capture.Multi Event DIO 11.Event 4":T8)  [unwired: 9 in]
    n117 = call "Capture Event.vi"("event # to capture"=T29 1 ("Settings.spark 3 shot 1"), "measured data"=w251) -> ("capture.<user name>"=→"capture.Multi Event DIO 12.Event 1":T8)  [unwired: 9 in]
    n118 = call "Capture Event.vi"("event # to capture"=T29 2 ("Settings.spark 3 shot 1"), "measured data"=w251) -> ("capture.<user name>"=→"capture.Multi Event DIO 12.Event 2":T8)  [unwired: 9 in]
    n119 = call "Capture Event.vi"("event # to capture"=T29 3 ("Settings.spark 3 shot 1"), "measured data"=w251) -> ("capture.<user name>"=→"capture.Multi Event DIO 12.Event 3":T8)  [unwired: 9 in]
    n120 = call "Capture Event.vi"("event # to capture"=T29 4 ("Settings.spark 3 shot 1"), "measured data"=w251) -> ("capture.<user name>"=→"capture.Multi Event DIO 12.Event 4":T8)  [unwired: 9 in]
    n121 = call "Capture Event.vi"("event # to capture"=T29 1 ("Settings.spark 4 shot 1"), "measured data"=w244) -> ("capture.<user name>"=→"capture.Multi Event DIO 13.Event 1":T8)  [unwired: 9 in]
    n122 = call "Capture Event.vi"("event # to capture"=T29 2 ("Settings.spark 4 shot 1"), "measured data"=w244) -> ("capture.<user name>"=→"capture.Multi Event DIO 13.Event 2":T8)  [unwired: 9 in]
    n123 = call "Capture Event.vi"("event # to capture"=T29 3 ("Settings.spark 4 shot 1"), "measured data"=w244) -> ("capture.<user name>"=→"capture.Multi Event DIO 13.Event 3":T8)  [unwired: 9 in]
    n124 = call "Capture Event.vi"("event # to capture"=T29 4 ("Settings.spark 4 shot 1"), "measured data"=w244) -> ("capture.<user name>"=→"capture.Multi Event DIO 13.Event 4":T8)  [unwired: 9 in]
    n125 = call "Capture Event.vi"("event # to capture"=T29 1 ("Settings.spark 5 shot 1"), "measured data"=w237) -> ("capture.<user name>"=→"capture.Multi Event DIO 14.Event 1":T8)  [unwired: 9 in]
    n126 = call "Capture Event.vi"("event # to capture"=T29 2 ("Settings.spark 5 shot 1"), "measured data"=w237) -> ("capture.<user name>"=→"capture.Multi Event DIO 14.Event 2":T8)  [unwired: 9 in]
    n127 = call "Capture Event.vi"("event # to capture"=T29 3 ("Settings.spark 5 shot 1"), "measured data"=w237) -> ("capture.<user name>"=→"capture.Multi Event DIO 14.Event 3":T8)  [unwired: 9 in]
    n128 = call "Capture Event.vi"("event # to capture"=T29 4 ("Settings.spark 5 shot 1"), "measured data"=w237) -> ("capture.<user name>"=→"capture.Multi Event DIO 14.Event 4":T8)  [unwired: 9 in]
    n129 = call "Capture Event.vi"("event # to capture"=T29 1 ("Settings.spark 6 shot 1"), "measured data"=w230) -> ("capture.<user name>"=→"capture.Multi Event DIO 15.Event 1":T8)  [unwired: 9 in]
    n130 = call "Capture Event.vi"("event # to capture"=T29 2 ("Settings.spark 6 shot 1"), "measured data"=w230) -> ("capture.<user name>"=→"capture.Multi Event DIO 15.Event 2":T8)  [unwired: 9 in]
    n131 = call "Capture Event.vi"("event # to capture"=T29 3 ("Settings.spark 6 shot 1"), "measured data"=w230) -> ("capture.<user name>"=→"capture.Multi Event DIO 15.Event 3":T8)  [unwired: 9 in]
    n132 = call "Capture Event.vi"("event # to capture"=T29 4 ("Settings.spark 6 shot 1"), "measured data"=w230) -> ("capture.<user name>"=→"capture.Multi Event DIO 15.Event 4":T8)  [unwired: 9 in]
  }
  n133 = node-c288(w16) -> ()
  n134 = node-c288(w14) -> ()
